vi "testInvKinematics.vi"() -> ()   [LabVIEW 2014]
uses:
  ICRMKinematics.llb/jntLims.ctl
  ICRMKinematics.llb/nloptIKParams.ctl
  ICRMKinematics.llb/knPms6A.ctl
  ICRMKinematics.llb/knPms11A.ctl
panel:
  in  "tabFK":enum32{"FK6A", "FK11A"}(tab)=enum."FK11A"
  in  "tab6A":T1(tab)
  out "H01":dbl[][](array[numeric])=[[0.955336489125606, 0.29404383655185584, -0.029502791919178276, 814.0], [-0.2955202066613396, 0.9505637859220634, -0.09537450575679464, -159.0], [0.0, 0.09983341664682814, 0.9950041652780258, -8.3], [0.0, 0.0, 0.0, 1.0]]
  out "H02":dbl[][](array[numeric])=[[0.8778758713520297, 0.47797859760337413, -0.029502791919178276, 814.0], [-0.4784773488526718, 0.8729049949946248, -0.09537450575679464, -159.0], [-0.01983383807620987, 0.0978433950072557, 0.9950041652780258, -8.3], [0.0, 0.0, 0.0, 1.0]]
  out "H03":dbl[][](array[numeric])=[[0.8778758713520297, 0.4479117241465462, -0.16943742759491745, 821.1985821450867], [-0.4784773488526718, 0.8057328996068985, -0.3490758099983131, -162.9235142605919], [-0.01983383807620987, 0.38751720202221734, 0.9216490856090721, -8.462637472224921], [0.0, 0.0, 0.0, 1.0]]
  out "H04":dbl[][](array[numeric])=[[-0.8058812194634177, -0.5673150960852107, -0.16943742759491745, 856.0547029730436], [0.5873940184440445, -0.7301467975483966, -0.3490758099983131, -110.1916446582601], [0.07432178154694849, -0.38084017091642125, 0.9216490856090721, 17.917632332001673], [0.0, 0.0, 0.0, 1.0]]
  out "H05":dbl[][](array[numeric])=[[-0.8058812194634177, -0.5673150960852107, -0.16943742759491745, 751.2901444427994], [0.5873940184440445, -0.7301467975483966, -0.3490758099983131, -33.83042226053432], [0.07432178154694849, -0.38084017091642125, 0.9216490856090721, 27.579463933104975], [0.0, 0.0, 0.0, 1.0]]
  out "ret_nl_pt":i32(ring)=3 items=["forced stop"=-5, "roundoff limited"=-4, "out of memory"=-3, "invalid args"=-2, "general failure"=-1, "zero shouldn't occur"=0, "success"=1, "error below errTol"=2, "function step tol reached"=3, "x step tol reached"=4, "max fun evals"=5, "max time"=6]
  out "xyz_nl_pt":dbl[](array[numeric])=[751.2901409187167, -33.83042383949764, 27.579460222970326]
  out "qps_nl_pt":dbl[](array[numeric])=[-0.6670053684228351, 0.6604166853963161, 0.7143005387100212, 2.445676128328102, 99.85960564414032]
  out "ret_nl_ptcs":i32(ring)=2 items=["forced stop"=-5, "roundoff limited"=-4, "out of memory"=-3, "invalid args"=-2, "general failure"=-1, "zero shouldn't occur"=0, "success"=1, "error below errTol"=2, "function step tol reached"=3, "x step tol reached"=4, "max fun evals"=5, "max time"=6]
  out "xyz_nl_ptcs":dbl[](array[numeric])=[751.5920711642107, -33.77244576793178, 27.690268477577728]
  out "qps_nl_ptcs":dbl[](array[numeric])=[-0.6666666666666666, 0.6584362139917697, 0.716049382716049, 2.4456412894375856, 99.79423868312757]
  out "ret_nl_ptppcs":i32(ring)=3 items=["forced stop"=-5, "roundoff limited"=-4, "out of memory"=-3, "invalid args"=-2, "general failure"=-1, "zero shouldn't occur"=0, "success"=1, "error below errTol"=2, "function step tol reached"=3, "x step tol reached"=4, "max fun evals"=5, "max time"=6]
  out "xyz_nl_ptppcs":dbl[](array[numeric])=[751.2902490221595, -33.82883491942012, 27.5784042479845]
  out "qps_nl_ptppcs":dbl[](array[numeric])=[-0.6669677348943719, 0.6603750933781924, 0.7142768435254334, 2.4456789154393435, 99.86103819614972]
  out "pp_nl_ptppcs":dbl[](array[numeric])=[0.39470809314068434, 2.6337659237235185]
  out "cs_nl_ptppcs":dbl[](array[numeric])=[0.4005414905452757, 21.74275851018672] caption="csGoal"
  in  "qpsLast":dbl[](array[numeric])=[0.0, 0.0, 0.0, 1.0, 10.0]
  out "ret_nl_ptmin":i32(ring)=3 items=["forced stop"=-5, "roundoff limited"=-4, "out of memory"=-3, "invalid args"=-2, "general failure"=-1, "zero shouldn't occur"=0, "success"=1, "error below errTol"=2, "function step tol reached"=3, "x step tol reached"=4, "max fun evals"=5, "max time"=6]
  out "xyz_nl_ptmin":dbl[](array[numeric])=[751.2901409187167, -33.83042383949764, 27.579460222970326]
  out "qps_nl_ptmin":dbl[](array[numeric])=[-0.6670053684228351, 0.6604166853963161, 0.7143005387100212, 2.445676128328102, 99.85960564414032]
  in  "kinematicParams":T2={"cathL"=103.0, "Rz01"=-0.3, "Tx01"=814.0, "Ty01"=-159.0, "Tz01"=-8.3, "Tx23"=8.2} {"Tx23" step=0.1; "Tz01" step=1.0; "Ty01" step=1.0; "Tx01" step=1.0; "Rz01" step=0.01; "cathL" step=1.0}
  out "xyzGoal":dbl[](array[numeric])=[751.2901444427994, -33.83042226053432, 27.579463933104975]
  out "ppGoal":dbl[](array[numeric])=[0.07439037439164771, 2.511743240918139]
  out "cs(goal)":dbl[](array[numeric])=[0.10598678097969841, 35.67202673868107] caption="csGoal"
  in  "tab11":enum32{"xyzpp", "Page 2"}(tab)
  out "qpsCnv":dbl[](array[numeric])=[0.08505930103247583, 0.4523249053046341, 0.1936583741186697, 2.4456412894375856, 101.39084112817793]
  out "ppCnv":dbl[](array[numeric])=[0.1430014613271996, 2.6783543659242044]
  out "xyzCnv":dbl[](array[numeric])=[734.3622410227802, 52.528415133991956, 6.599511271324888]
  in  "kn0":T3={"tx01"=806.0, "ty01"=-66.0, "tz01"=-28.0, "ry01"=0.0, "rz01"=-0.24, "tx23"=8.2, "ry34"=0.0, "rz34"=0.0, "cathL"=98.0, "ry45"=0.0, "rz45"=0.0}
  out "xyz11Goal":dbl[](array[numeric])=[734.3618148529447, 52.52735088036842, 6.598868311540576]
  out "pp11Goal":dbl[](array[numeric])=[0.07439037439164772, 2.571743240918139]
  out "err_nl_ptmin":errorcluster
  out "err_nl_ptppcs":errorcluster
  in  "qpsInit":dbl[](array[numeric])=[0.0, 0.0, 0.0, 1.0, 10.0]
  out "err_nl_ptcs":errorcluster
  out "err_nl_pt":errorcluster
  in  "jntLims":T4={"dn"=[-3.0, -0.8, -1.0, 0.001, 0.0], "up"=[3.0, 0.8, 1.0, 5.0, 500.0]}
  in  "nlParams":T5={"maxIts"=10000.0, "maxTimeSec"=1.0, "nlMethod"=enum."GN_DIRECT", "errTol"=1e-06, "tolFun"=1e-06, "tolX"=1e-06}
  in  "qpsGoal":dbl[](array[numeric])=[0.1, -0.2, 0.3, 3.0, 130.0]
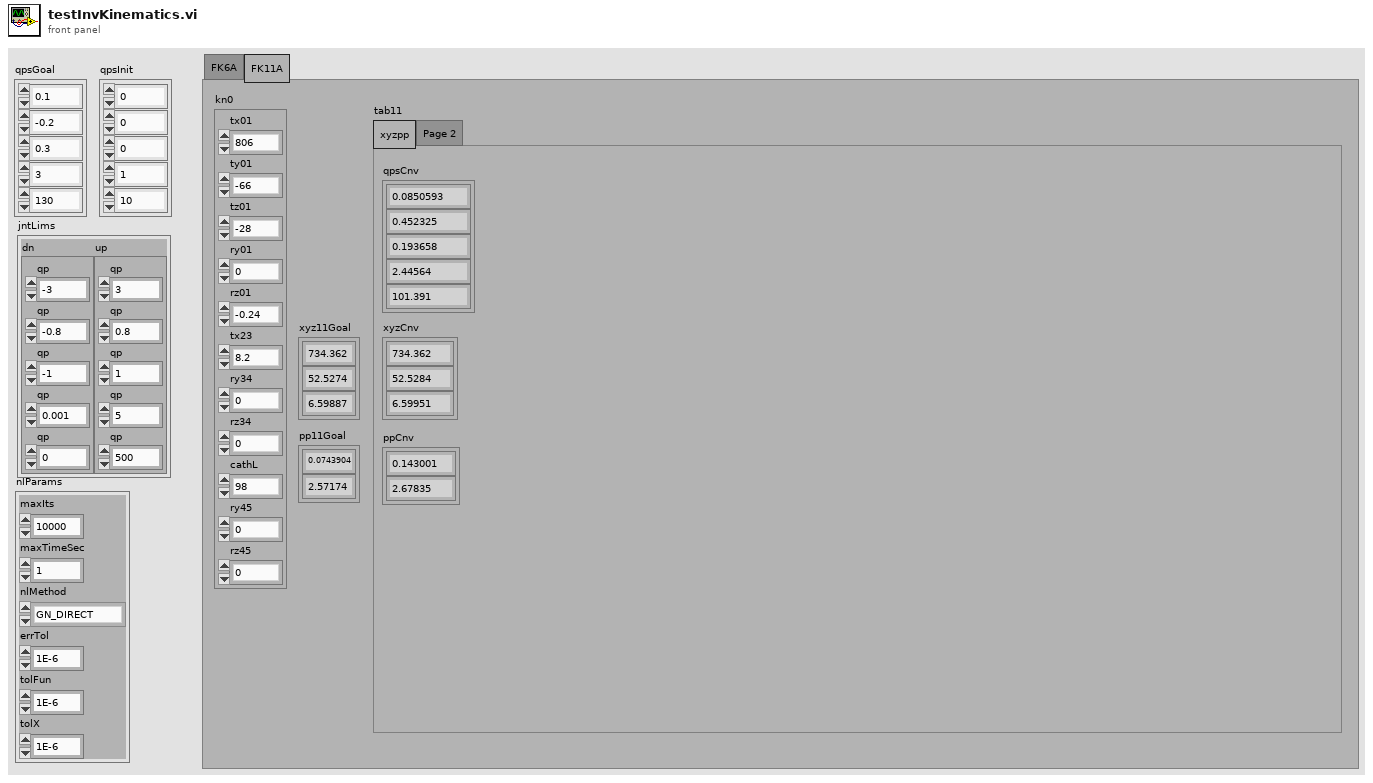
[diagram p1: front panel]
types:
  T1 = enum32{"getH", "NR", "xyz", "xyzcs", "xyzppcs", "xyzMin", "xyzKal"}
  T2 = typedef "knPms6A.ctl" = cluster{"cathL":dbl, "Rz01":dbl, "Tx01":dbl, "Ty01":dbl, "Tz01":dbl, "Tx23":dbl}
  T3 = typedef "knPms11A.ctl" = cluster{"tx01":dbl, "ty01":dbl, "tz01":dbl, "ry01":dbl, "rz01":dbl, "tx23":dbl, "ry34":dbl, "rz34":dbl, "cathL":dbl, "ry45":dbl, "rz45":dbl}
  T4 = typedef "jntLims.ctl" = cluster{"dn":dbl[], "up":dbl[]}
  T5 = typedef "nloptIKParams.ctl" = cluster{"maxIts":dbl, "maxTimeSec":dbl, "nlMethod":enum16{"GN_DIRECT", "GN_DIRECT_L", "GN_DIRECT_L_NOSCAL", "GN_DIRECT_L_RAND", "GN_DIRECT_L_RAND_NOSCAL", "GN_DIRECT_NOSCAL", "GN_ESCH", "GN_ISRES", "GN_MLSL", "GN_MLSL_LDS", "GN_ORIG_DIRECT", "GN_ORIG_DIRECT_L", "LN_BOBYQA", "LN_COBYLA", "LN_NELDERMEAD", "LN_NEWUOA", "LN_NEWUOA_BOUND", "LN_PRAXIS", "LN_SBPLX"}, "errTol":dbl, "tolFun":dbl, "tolX":dbl}
  T6 = cluster{"kinematicParams":T2, "nlParams":T5, "jntLims":T4}
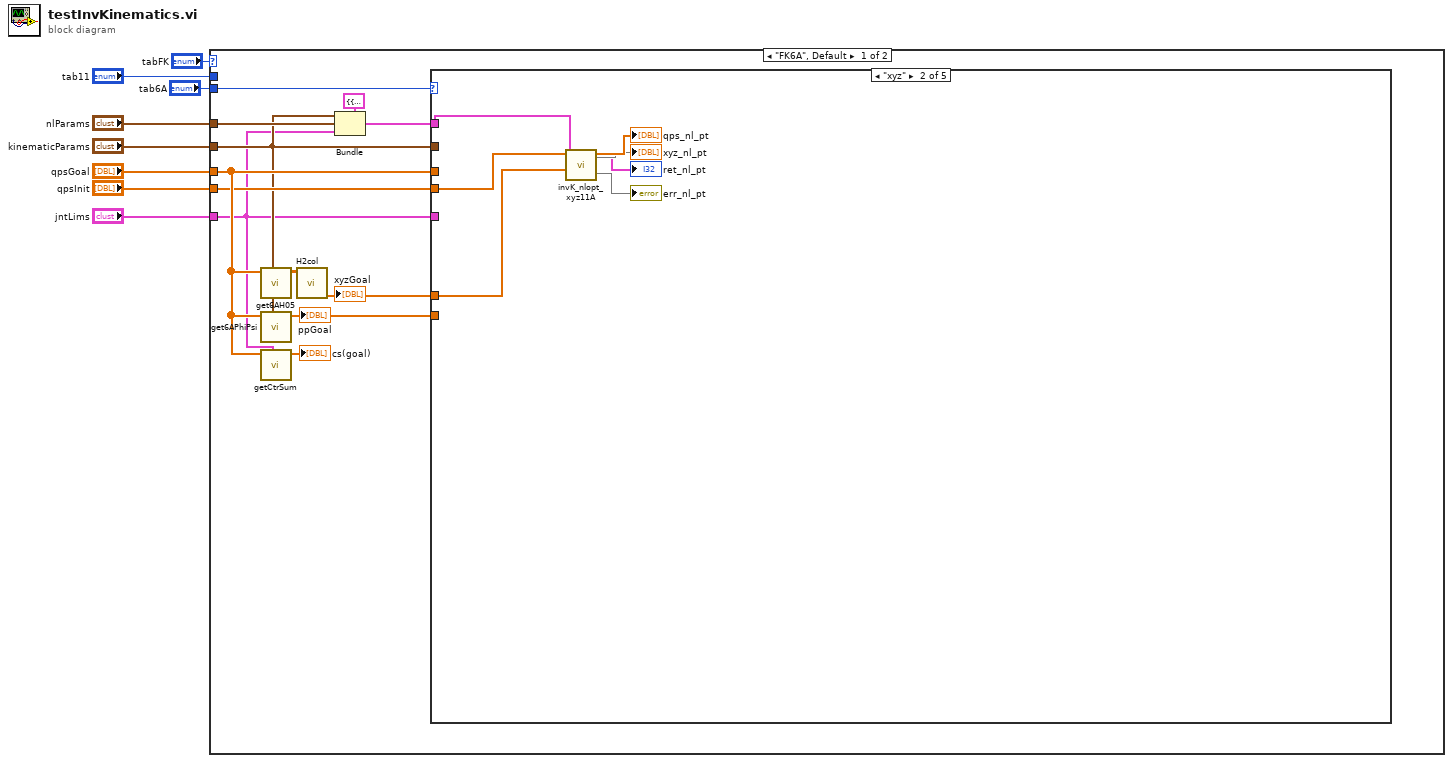
[diagram p0: block diagram]
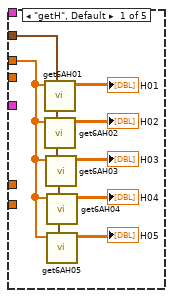
[diagram p2: hidden frame]
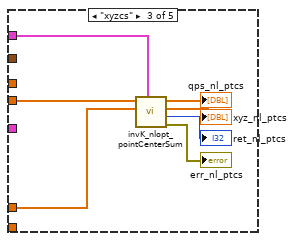
[diagram p3: hidden frame]
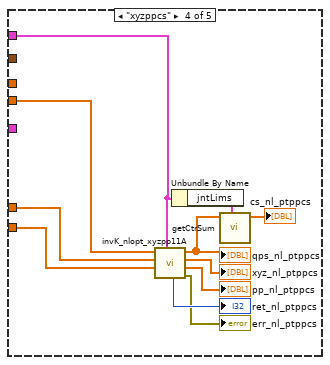
[diagram p4: hidden frame]
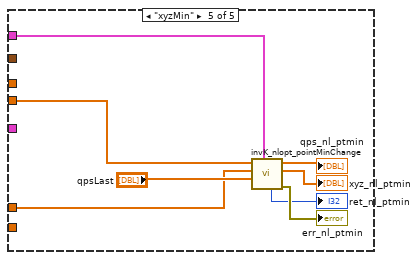
[diagram p5: hidden frame]
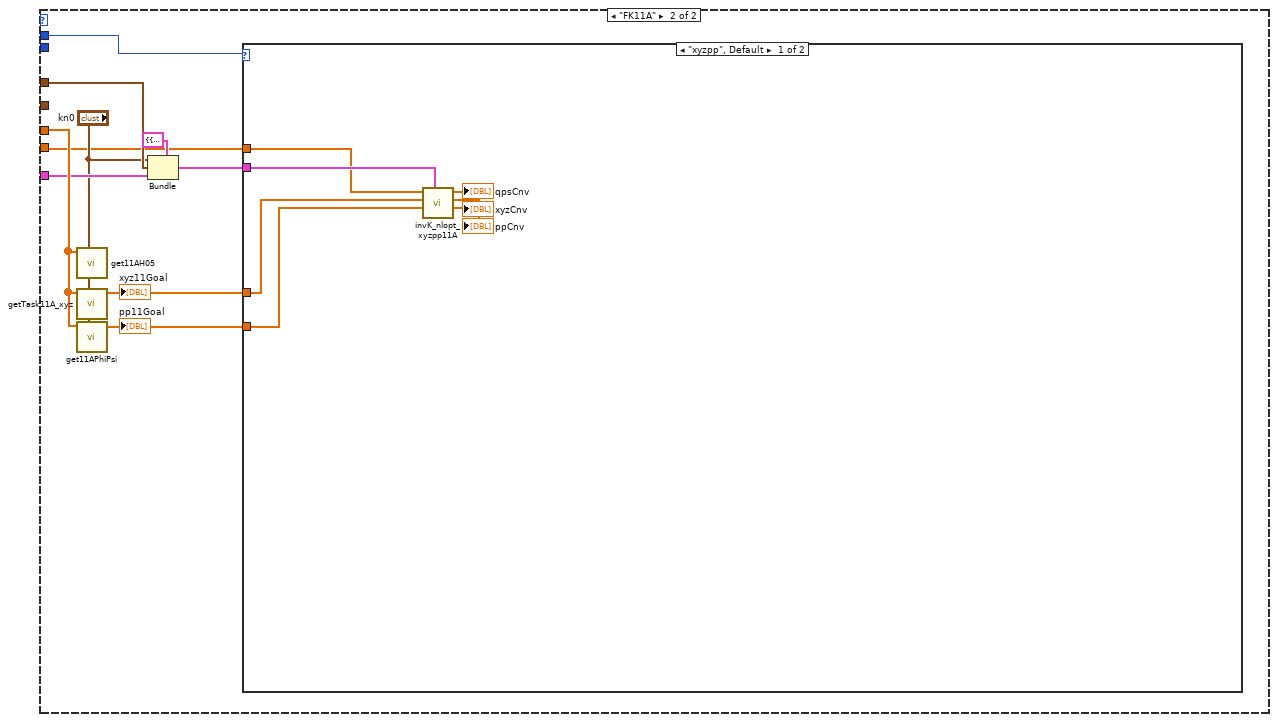
[diagram p6: hidden frame]
diagram:
  n1 = case shown="\"FK6A\", Default" "tabFK" {
    tunnel: "tab6A" -> [w20 _]
    tunnel: "kinematicParams" -> [w11 _]
    tunnel: "qpsGoal" -> [w17 w68]
    tunnel: "jntLims" -> [w10 w67]
    tunnel: "qpsInit" -> [w16 w63]
    tunnel: "nlParams" -> [w12 w66]
    tunnel: "tab11" -> [_ w70]
    frame "FK6A", Default {
      n2 = call "get6AH05.vi"("kinematicParams"=w11, "qps"=w17) -> ("H05"=w18:dbl[][])  [unwired: 9 in]
      n3 = call "get6APhiPsi.vi"("knParams"=w11, "qp0"=w17) -> ("pp"=w14:dbl[])  [unwired: 7 in, 2 out]
      "ppGoal" <- w14
      n4 = call "getCtrSum.vi"("jntLims"=w10, "qp0"=w17) -> ("cs"=→"cs(goal)":dbl[])  [unwired: 7 in, 2 out]
      n5 = call "H2col.vi"("H"=w18) -> ("xyz"=w15:dbl[])  [unwired: 6 in, 4 out]
      "xyzGoal" <- w15
      n6 = Bundle(cluster=T6 {"kinematicParams"={"cathL"=95.0, "Rz01"=-0.4712, "Tx01"=766.6, "Ty01"=-112.0, "Tz01"=14.7, "Tx23"=8.2}, "nlParams"={"maxIts"=1000.0, "maxTimeSec"=1.0, "nlMethod"=enum."LN_BOBYQA", "errTol"=0.001, "tolFun"=0.001, "tolX"=0.001}, "jntLims"={"dn"=[-3.0, -0.8, -1.0, 0.001, 0.0], "up"=[3.0, 0.8, 1.0, 5.0, 500.0]}} ("nlCfg"), "kinematicParams"=w11, "nlParams"=w12, "jntLims"=w10) -> (w9:T6)
      n7 = case shown="\"xyz\"" w20 {
        tunnel: w11 -> [w22 _ _ _ _]
        tunnel: w17 -> [w21 _ _ _ _]
        tunnel: w16 -> [_ w29 w37 w42 w54]
        tunnel: w10 -> [_ _ _ _ _]
        tunnel: w15 -> [_ w28 w36 w44 w55]
        tunnel: w14 -> [_ _ _ w43 _]
        tunnel: w9 -> [_ w30 w35 w45 w53]
        frame "getH", Default {
          n8 = call "get6AH01.vi"("kinematicParams"=w22, "qps"=w21) -> ("H01"=→"H01":dbl[][])  [unwired: 9 in]
          n9 = call "get6AH02.vi"("kinematicParams"=w22, "qps"=w21) -> ("H02"=→"H02":dbl[][])  [unwired: 9 in]
          n10 = call "get6AH03.vi"("kinematicParams"=w22, "qps"=w21) -> ("H03"=→"H03":dbl[][])  [unwired: 9 in]
          n11 = call "get6AH04.vi"("kinematicParams"=w22, "qps"=w21) -> ("H04"=→"H04":dbl[][])  [unwired: 9 in]
          n12 = call "get6AH05.vi"("kinematicParams"=w22, "qps"=w21) -> ("H05"=→"H05":dbl[][])  [unwired: 9 in]
        }
        frame "xyz" {
          n13 = call "invK_nlopt_xyz11A.vi"(9:w28, "xyzGoal"=w30, "qp0"=w29) -> ("qpsCnv"=→"qps_nl_pt":dbl[], 5:→"xyz_nl_pt", 6:→"err_nl_pt", "pms"=→"ret_nl_pt":cluster{"kn":T3, "nlParams":T5, "jntLims":T4})  [unwired: 1 in, 4 out]
        }
        frame "xyzcs" {
          n14 = call "invK_nlopt_pointCenterSum.vi"("nlCfg"=w35, "xyzGoal"=w36, "qp0"=w37) -> ("error out"=→"err_nl_ptcs":errorcluster, "retCodeOut"=→"ret_nl_ptcs":i32, "xyzCnv"=→"xyz_nl_ptcs":dbl[], "qpsCnv"=→"qps_nl_ptcs":dbl[])  [unwired: 5 in]
        }
        frame "xyzppcs" {
          n15 = call "invK_nlopt_xyzpp11A.vi"("pms"=w45, "ppGoal"=w43, "xyzGoal"=w44, "qp0"=w42) -> ("error out"=→"err_nl_ptppcs":errorcluster, "ppCnv"=→"pp_nl_ptppcs":dbl[], "xyzCnv"=→"xyz_nl_ptppcs":dbl[], "qpsCnv"=w51:dbl[], "retCodeOut"=→"ret_nl_ptppcs":i32)  [unwired: 3 in]
          "qps_nl_ptppcs" <- w51
          n16 = Unbundle By Name(w45) -> ("jntLims"=w46:T4)
          n17 = call "getCtrSum.vi"("jntLims"=w46, "qp0"=w51) -> ("cs"=→"cs_nl_ptppcs":dbl[])  [unwired: 7 in, 2 out]
        }
        frame "xyzMin" {
          n18 = call "invK_nlopt_pointMinChange.vi"("nlCfg"=w53, "qpsLast"="qpsLast", "xyzGoal"=w55, "qp0"=w54) -> ("error out"=→"err_nl_ptmin":errorcluster, "xyzCnv"=→"xyz_nl_ptmin":dbl[], "qpsCnv"=→"qps_nl_ptmin":dbl[], "retCodeOut"=→"ret_nl_ptmin":i32)  [unwired: 4 in]
        }
      }
    }
    frame "FK11A" {
      n19 = call "get11AH05.vi"("kn0"="kn0", "qps"=w68) -> ()  [unwired: 9 in, 1 out]
      n20 = call "getTask11A_xyz.vi"("kn0"="kn0", "qps"=w68) -> ("xyz"=w62:dbl[])  [unwired: 9 in]
      "xyz11Goal" <- w62
      n21 = call "get11APhiPsi.vi"("kn0"="kn0", "qps"=w68) -> ("pp"=w61:dbl[])  [unwired: 9 in]
      "pp11Goal" <- w61
      n22 = Bundle(cluster=cluster{"kn0":T3, "nlParams":T5, "jntLims":T4} {"kn0"={"tx01"=0.0, "ty01"=0.0, "tz01"=0.0, "ry01"=0.0, "rz01"=0.0, "tx23"=0.0, "ry34"=0.0, "rz34"=0.0, "cathL"=0.0, "ry45"=0.0, "rz45"=0.0}, "nlParams"={"maxIts"=0.0, "maxTimeSec"=0.0, "nlMethod"=enum."GN_DIRECT", "errTol"=0.0, "tolFun"=0.0, "tolX"=0.0}, "jntLims"={"dn"=[], "up"=[]}} ("pms"), "kn0"="kn0", "nlParams"=w66, "jntLims"=w67) -> (w65:cluster{"kn0":T3, "nlParams":T5, "jntLims":T4})
      n23 = case shown="\"xyzpp\", Default" w70 {
        tunnel: w65 -> [w74 _]
        tunnel: w63 -> [w73 _]
        tunnel: w62 -> [w72 _]
        tunnel: w61 -> [w71 _]
        frame "xyzpp", Default {
          n24 = call "invK_nlopt_xyzpp11A.vi"("pms"=w74, "ppGoal"=w71, "xyzGoal"=w72, "qp0"=w73) -> ("ppCnv"=→"ppCnv":dbl[], "xyzCnv"=→"xyzCnv":dbl[], "qpsCnv"=→"qpsCnv":dbl[])  [unwired: 3 in, 2 out]
        }
        frame "Page 2" {
        }
      }
    }
  }
